vi "Switch Box Cell Select Control.vi"(0 "PhyChls":tag="Dev1/port1/line1:4", 1 "line grouping":i32(ring) items=["one channel for each line", "one channel for all lines"], 2 "Cell":i32, 5 "All OFF":bool, 7 "Dout Inv":bool[](array[boolean])=[FALSE, FALSE, FALSE, FALSE], 11 "ErrIn":errorcluster, 12 "SimOn":bool, 13 "Init":bool, 14 "Stop":bool) -> (15 "ErrOut":errorcluster)   [LabVIEW 2013]
uses:
  <vilib>/DAQmx/write.llb/DAQmx Write (Digital 1D Bool NChan 1Samp 1Line).vi
  <vilib>/DAQmx/create/channels.llb/DAQmx Create Channel (DO-Digital Output).vi
  <vilib>/DAQmx/miscellaneous.llb/DAQmx Fill In Error Info.vi
panel:
  out "x .xor. y?":bool[](array[boolean])
  # "ER2007"
  # "YCL1 -> YCL4"
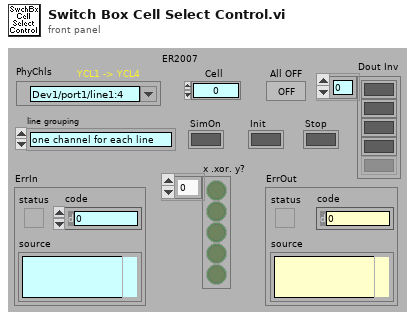
[diagram p1: front panel]
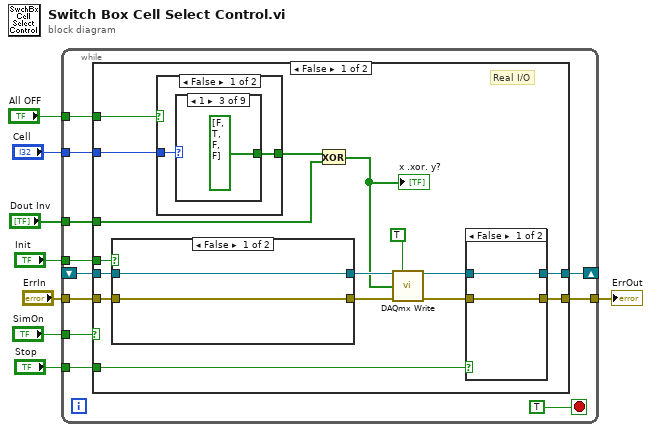
[diagram p0: block diagram]
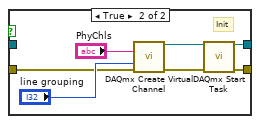
[diagram p2: hidden frame]
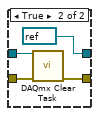
[diagram p3: hidden frame]
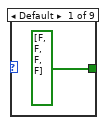
[diagram p4: hidden frame]
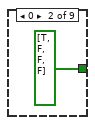
[diagram p5: hidden frame]
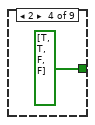
[diagram p6: hidden frame]
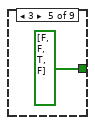
[diagram p7: hidden frame]
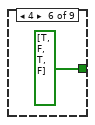
[diagram p8: hidden frame]
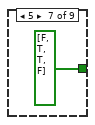
[diagram p9: hidden frame]
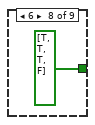
[diagram p10: hidden frame]
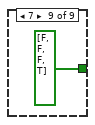
[diagram p11: hidden frame]
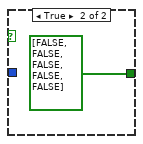
[diagram p12: hidden frame]
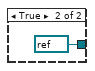
[diagram p14: hidden frame]
diagram:
  n1 = while {
    tunnel: "ErrIn" -> [w19]
    tunnel: [w18] -> w7
    tunnel: "SimOn" -> [w17]
    tunnel: "Stop" -> [w15]
    shift-right: [w14] -> _
    shift-left: _ -> [w12]
    tunnel: "Init" -> [w13]
    tunnel: "All OFF" -> [w11]
    tunnel: "Cell" -> [w10]
    tunnel: "Dout Inv" -> [w9]
    stop <- TRUE stop-if-true
    n2 = case shown="False" w17 {
      tunnel: w19 -> [w35 w66]
      tunnel: [w29 w66] -> w18
      tunnel: w15 -> [w26 _]
      tunnel: [w25 w63] -> w14
      tunnel: w13 -> [w24 w65]
      tunnel: w12 -> [w23 w64]
      tunnel: w11 -> [w22 _]
      tunnel: w10 -> [w21 _]
      tunnel: w9 -> [w20 _]
      frame False {
        # "Real I/O"
        n3 = case shown="False" w24 {
          tunnel: w35 -> [w36 w42]
          tunnel: [w36 w38] -> w34
          tunnel: [w37 w39] -> w33
          tunnel: w23 -> [w37 _]
          frame False {
          }
          frame True {
            # "Init"
            n4 = call-poly <vilib>:"DAQmx Create Virtual Channel.vi"("lines"="PhyChls", "line grouping"="line grouping", "error in"=w42) -> ("task out"=w40:refnum<k21>, "error out"=w41:errorcluster)  [unwired: 11 in]
            n5 = call <vilib>:"DAQmx Start Task.vi"("task/channels in"=w40, "error in"=w41) -> ("task out"=w39:refnum<k21>, "error out"=w38:errorcluster)  [unwired: 12 in]
          }
        }
        n6 = case shown="False" w22 {
          tunnel: [w51 bool[] [FALSE, FALSE, FALSE, FALSE, FALSE]] -> w28
          tunnel: w21 -> [w52 _]
          frame False {
            n7 = case shown="1" w52 {
              tunnel: [bool[] [FALSE, FALSE, FALSE, FALSE] bool[] [TRUE, FALSE, FALSE, FALSE] bool[] [FALSE, TRUE, FALSE, FALSE] bool[] [TRUE, TRUE, FALSE, FALSE] bool[] [FALSE, FALSE, TRUE, FALSE] bool[] [TRUE, FALSE, TRUE, FALSE] bool[] [FALSE, TRUE, TRUE, FALSE] bool[] [TRUE, TRUE, TRUE, FALSE] bool[] [FALSE, FALSE, FALSE, TRUE]] -> w51
              frame Default {
              }
              frame 0 {
              }
              frame 1 {
              }
              frame 2 {
              }
              frame 3 {
              }
              frame 4 {
              }
              frame 5 {
              }
              frame 6 {
              }
              frame 7 {
              }
            }
          }
          frame True {
          }
        }
        n8 = Exclusive Or(1:w20, 2:w28) -> (0:w27:bool[])
        "x .xor. y?" <- w27
        n9 = call-poly <vilib>:"DAQmx Write.vi"("task/channels in"=w33, "auto start"=TRUE, "data"=w27, "error in"=w34) -> ("task out"=w30:refnum<k21>, "error out"=w31:errorcluster)  [unwired: 9 in, 1 out]
        n10 = case shown="False" w26 {
          tunnel: w31 -> [w46 w50]
          tunnel: w30 -> [w45 w49]
          tunnel: [w46 w48] -> w29
          tunnel: [w45 refnum<k21> refnum ("task out")] -> w25
          frame False {
          }
          frame True {
            n11 = call <vilib>:"DAQmx Clear Task.vi"("task in"=w49, "error in"=w50) -> ("error out"=w48:errorcluster)  [unwired: 13 in]
          }
        }
      }
      frame True {
        # "Simulation"
        n12 = case shown="False" w65 {
          tunnel: w64 -> [w67 _]
          tunnel: [w67 refnum<k21> refnum ("task out")] -> w63
          frame False {
          }
          frame True {
          }
        }
      }
    }
  }
  "ErrOut" <- w7
